vi "template-json-interface.vi"() -> ()   [LabVIEW 2024]
uses:
  template-state-machine-iwh/state-enum.ctl
  utils-sub-vi/csv-file-logging-util/filepath-selection.ctl
  utils-sub-vi/csv-file-logging-util/datalogging-options.ctl
  template-state-machine-iwh/serial-options.ctl
  template-state-machine-iwh/sensor-options.ctl
  <vilib>/Instr/_visa.llb/VISA Configure Serial Port (Instr).vi
  arduino-serial-ctrl.ctl
panel:
  out "Units":string
  out "Data":dbl
  out "Data Plot Chart":dbl(graph)
  out "Serial Port Open":bool
  out "Log File Open":bool
  in  "Tab Control":enum32{"Run", "Settings"}(tab)
  out "Logged CSV out":string
  out "Serial msg":string
  in  "Datalogging options":T1={"data-precision"=3, "Include Date"=FALSE, "Include Timestamp"=TRUE, "Include Milliseconds"=FALSE, "sample-rate (Hz)"=4.0, "Logging Active"=TRUE}
  in  "Log Filepath Selection":T2={"Log Filepath Source"=enum."Application Relative (Auto)", "Log File Path (Manual)"=path "C:/Users/dheard/Documents/0002-labview-projects/adam-4xxx/template/data", "Log File Folder Name"="data", "log file name"="log", "Include Date in Filename"=TRUE, "Include Time in Filename"=TRUE}
  in  "Serial Port Options":T3={"COM Port "="COM29", "baud rate (115200)"=115200, "Simulate Hardware"=FALSE} {"baud rate (115200)" max=115200 step=1200}
  in  "Sensor Options":T4={"Display Units"="PSI", "Zero Offset"=2.62, "Sensor Min"=0.0, "Sensor Max"=500.0, "Signal Min"=0.0, "Signal Max"=100.0, "Conversion Factor"=0.0}
  in  "save-settings":bool
  in  "load-settings":bool
  in  "Settings file":path=path "C:/Users/dheard/Documents/0002-labview-projects/labview-template-state-machine/settings/arduino-json-config.ini"
  out "Sample Rate (Hz)":dbl format="%-#3.3f"
  in  "Debug Mode":bool
  out "Loop Time (mS)":u32
  out "State:":T5
  out "error IO":errorcluster
  in  "stop":bool
  in  "start":bool
  in  "Exit":bool
  # "Arduino JSON Interface"
  # "Live Data"
  # "Conversion Factor to\nCalculate User Units from Sensor Units"
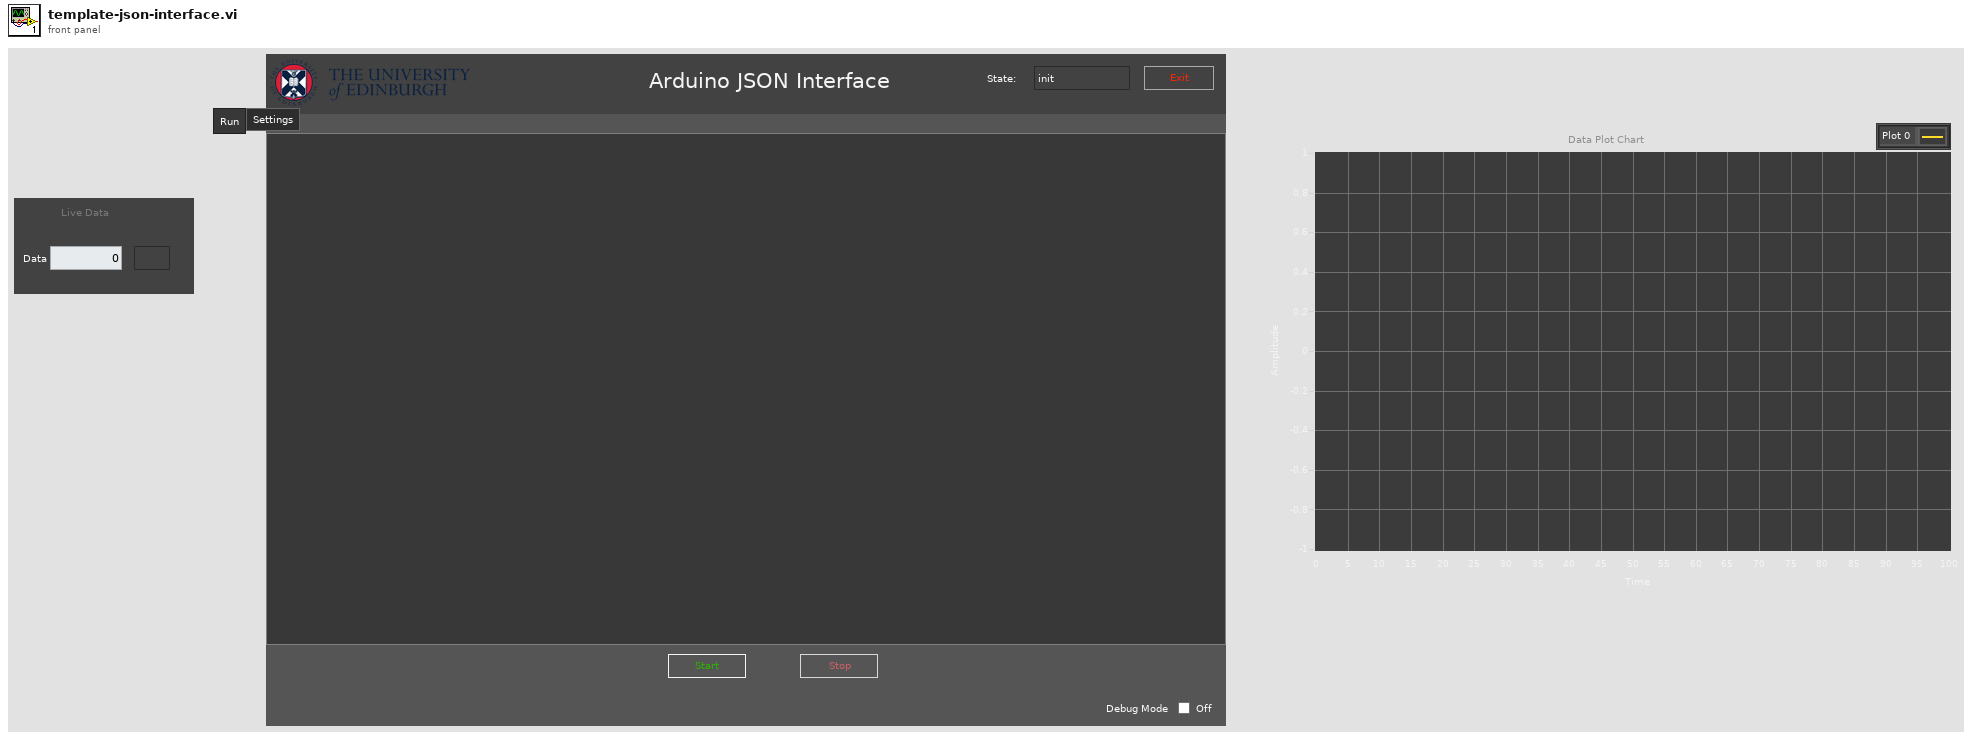
[diagram p1: front panel]
types:
  T1 = typedef "datalogging-options.ctl" = cluster{"data-precision":i32, "Include Date":bool, "Include Timestamp":bool, "Include Milliseconds":bool, "sample-rate (Hz)":dbl, "Logging Active":bool}
  T2 = typedef "filepath-selection.ctl" = cluster{"Log Filepath Source":enum16{"Application Relative (Auto)", "VI Relative (Auto)", "Complete Path (Manual)"}, "Log File Path (Manual)":path, "Log File Folder Name":string, "log file name":string, "Include Date in Filename":bool, "Include Time in Filename":bool}
  T3 = typedef "arduino-serial-ctrl.ctl" = cluster{"COM Port ":refnum<visa-resource-name>, "baud rate (115200)":u32, "Simulate Hardware":bool}
  T4 = typedef "sensor-options.ctl" = cluster{"Display Units":string, "Zero Offset":dbl, "Sensor Min":dbl, "Sensor Max":dbl, "Signal Min":dbl, "Signal Max":dbl, "Conversion Factor":dbl}
  T5 = typedef "state-enum.ctl" = enum16{"init", "recall-settings", "save-settings", "wait", "start", "pre-run", "run", "stop", "shutdown", "exit"}
  T6 = typedef "serial-options.ctl" = cluster{"COM Port (COM10)":refnum<visa-resource-name>, "baud rate (19200)":u32, "Simulate Hardware":bool}
  T7 = enum8{"Enabled", "Disabled", "Disabled and Grayed Out"}
  T8 = enum16{"open", "replace", "create", "open or create", "replace or create", "replace or create with confirmation"}
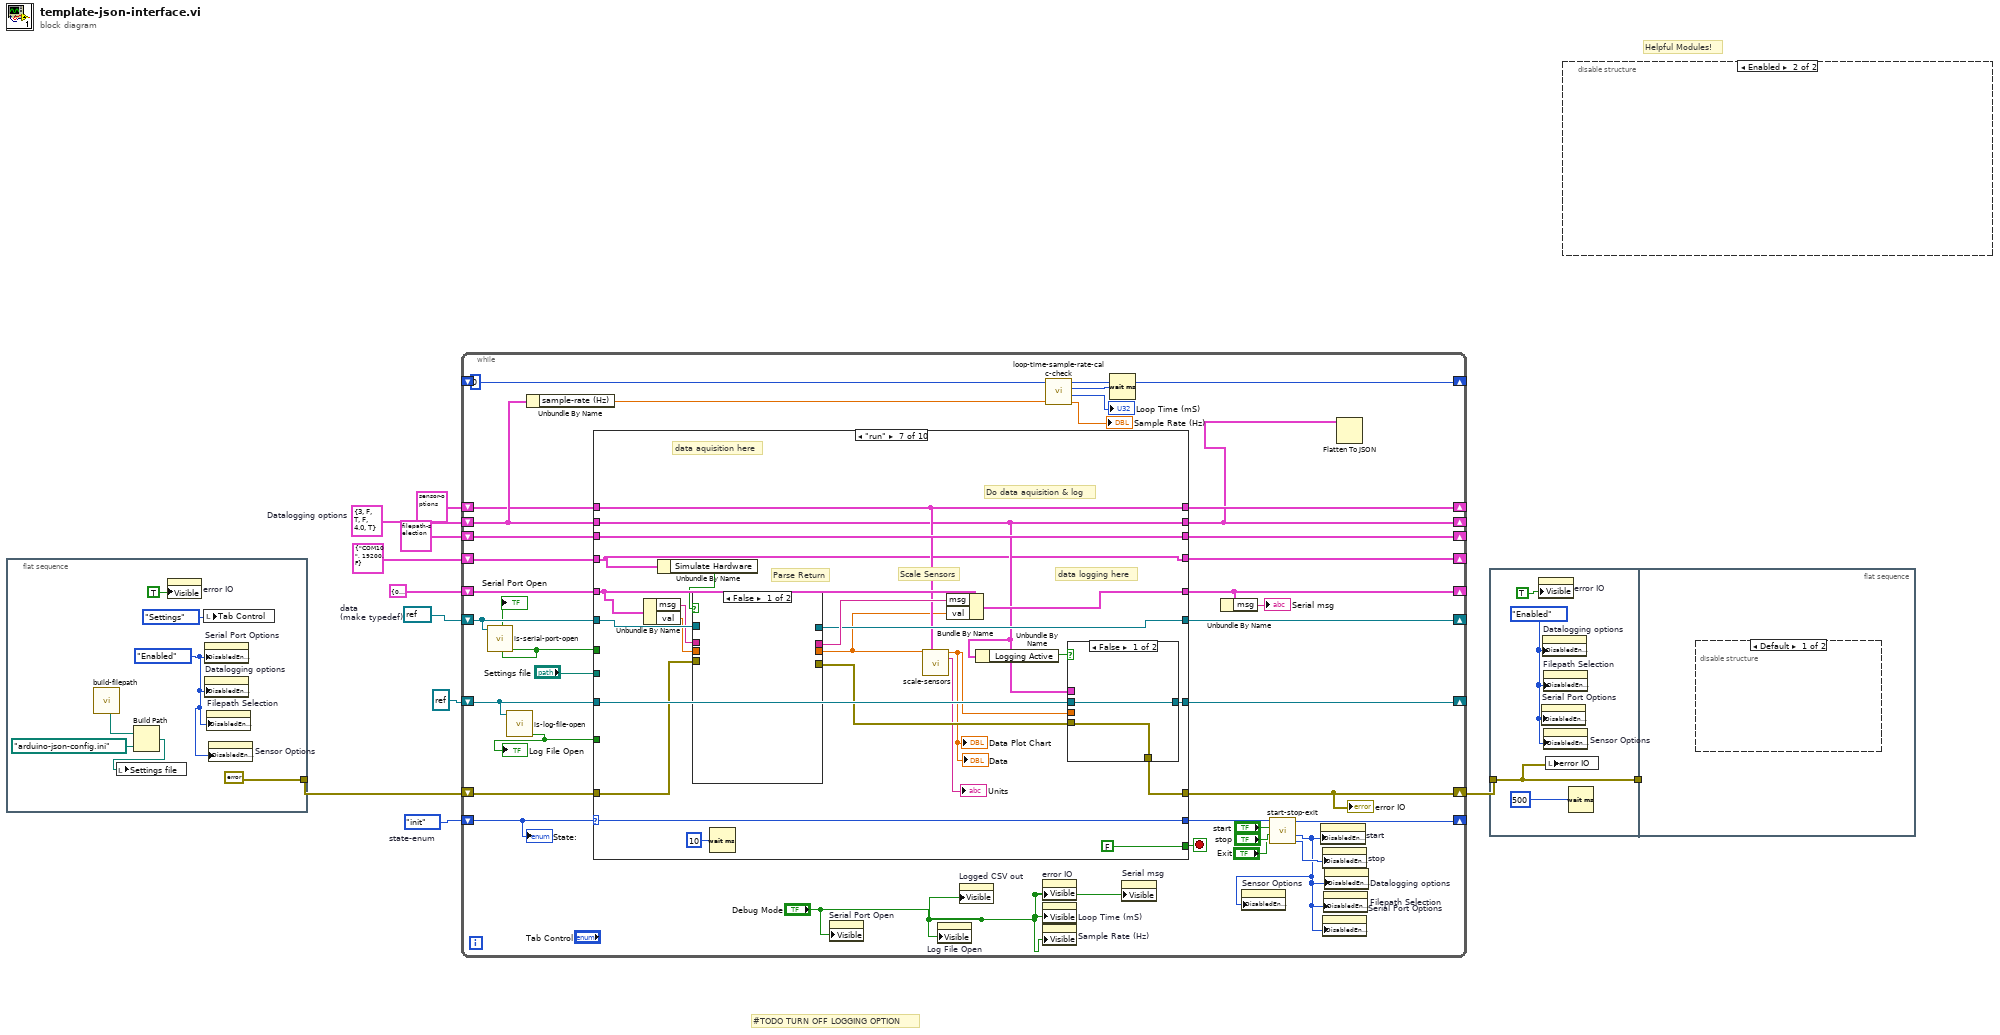
[diagram p0: block diagram]
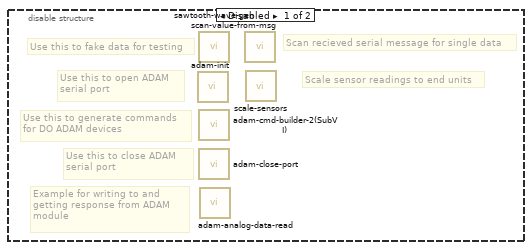
[diagram p2: hidden frame]
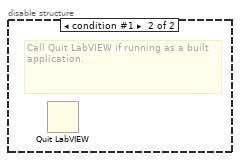
[diagram p3: hidden frame]
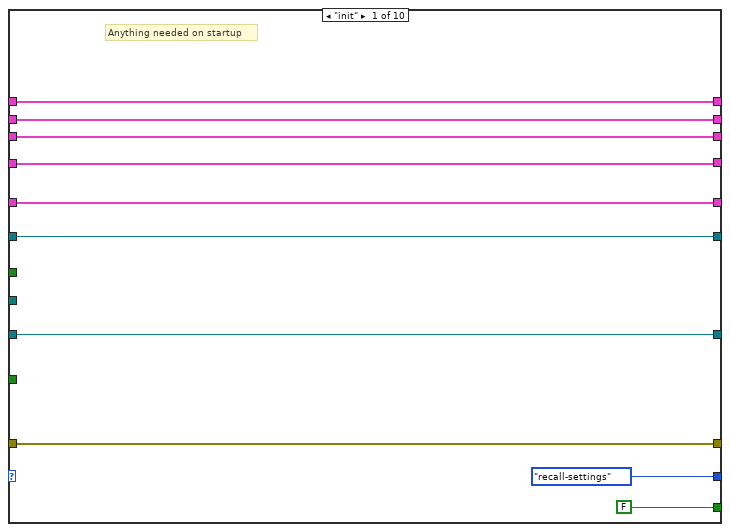
[diagram p4: hidden frame]
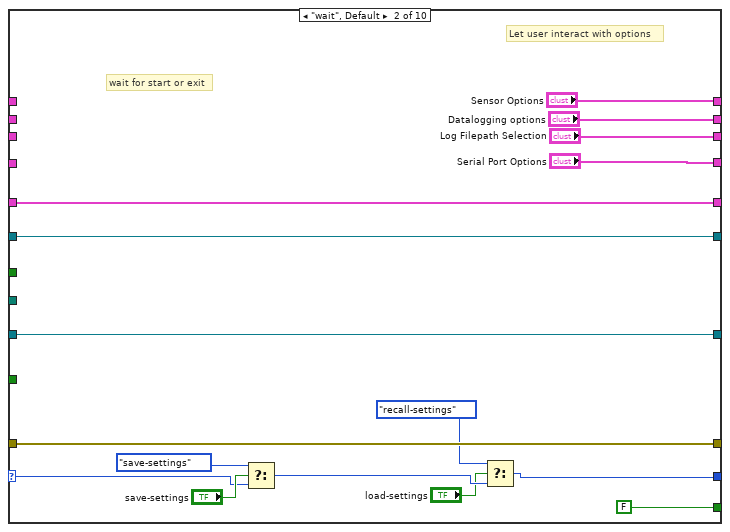
[diagram p5: hidden frame]
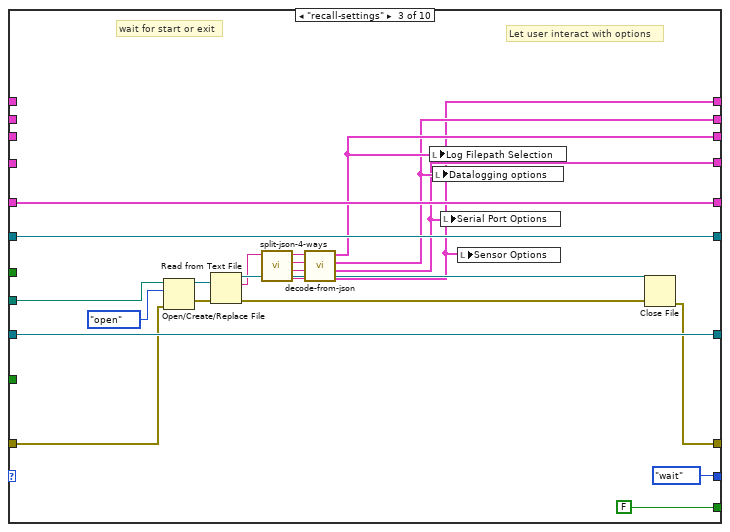
[diagram p6: hidden frame]
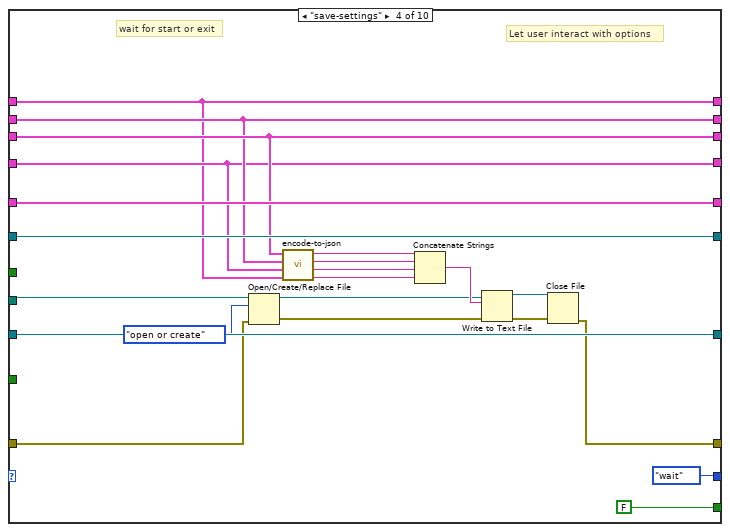
[diagram p7: hidden frame]
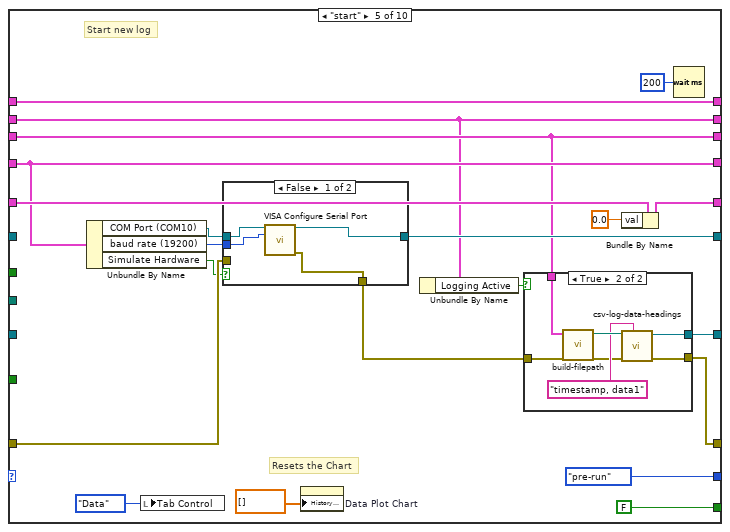
[diagram p8: hidden frame]
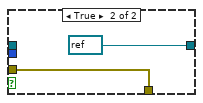
[diagram p9: hidden frame]
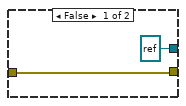
[diagram p10: hidden frame]
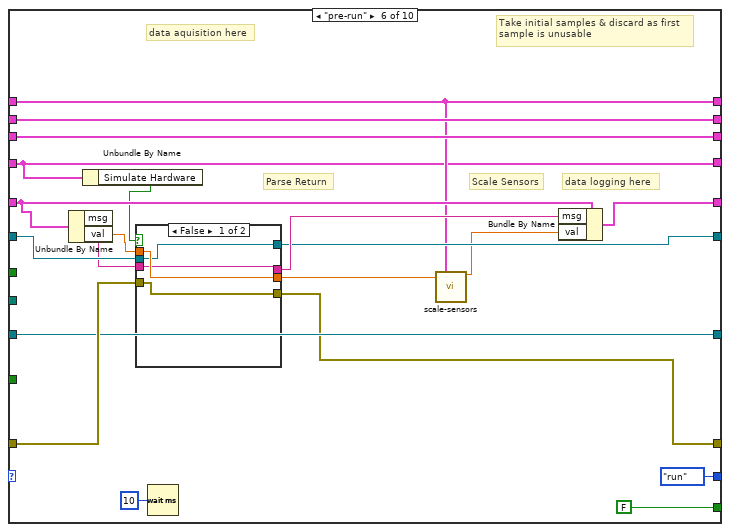
[diagram p11: hidden frame]
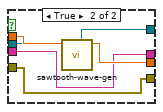
[diagram p12: hidden frame]
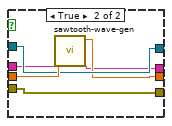
[diagram p13: hidden frame]
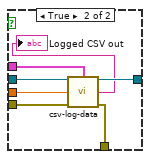
[diagram p14: hidden frame]
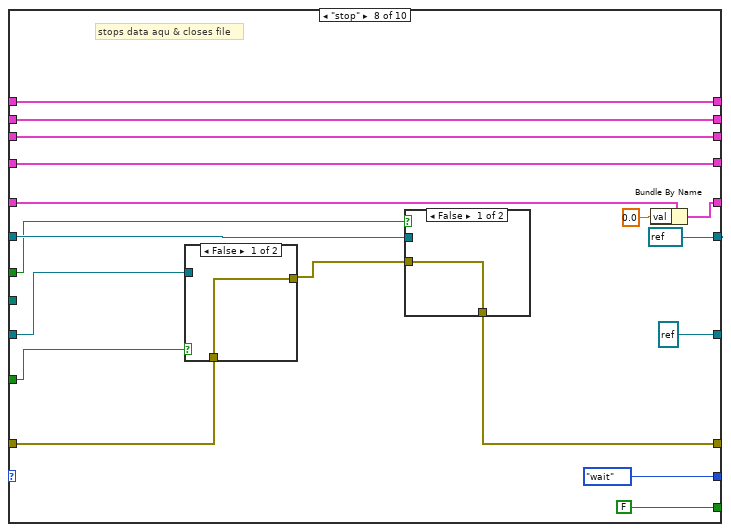
[diagram p15: hidden frame]
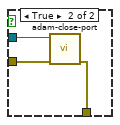
[diagram p16: hidden frame]
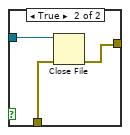
[diagram p17: hidden frame]
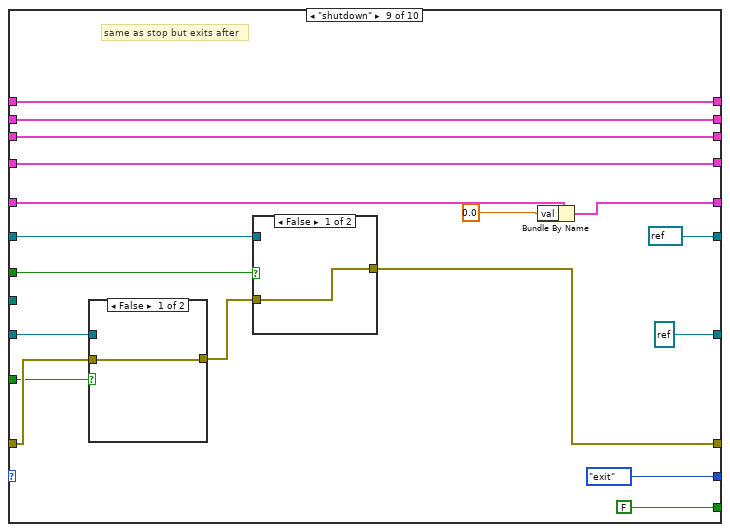
[diagram p18: hidden frame]
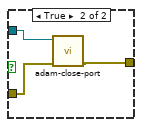
[diagram p19: hidden frame]
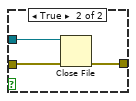
[diagram p20: hidden frame]
diagram:
  w4 = T1 {"data-precision"=3, "Include Date"=FALSE, "Include Timestamp"=TRUE, "Include Milliseconds"=FALSE, "sample-rate (Hz)"=4.0, "Logging Active"=TRUE}  # Datalogging options
  w9 = cluster{"val":dbl, "bool":bool, "msg":string} {"val"=0.0, "bool"=FALSE, "msg"=""}  # data (make typedef)
  w12 = state-enum."init"  # state-enum
  # "#TODO TURN OFF LOGGING OPTION"
  # "Helpful Modules!"
  n1 = flat-sequence {
    tunnel: [errorcluster {"status"=FALSE, "code"=0, "source"=""} ("error IO")] -> w8
    frame #0 {
      w16 = T7."Enabled" ("Disabled")
      n2 = call "build-filepath.vi"() -> ("Application Directory"=w15:path)  [unwired: 9 in, 2 out]
      n3 = Build Path(base path=w15, name or relative path=path "arduino-json-config.ini") -> (appended path=w13:path)
      n4 = local write "Settings file"(w13) -> ()
      n5 = property on="error IO" class="Clust (strict)"("Visible"=TRUE) -> ()  [unwired: 2 in, 2 out]
      n6 = local write "Tab Control"(enum32{"Data", "Settings"}."Settings" ("Tab Control")) -> ()
      n7 = property on="Serial Port Options" class="Clust (strict)"("DisabledEnum"=w16) -> ()  [unwired: 2 in, 2 out]
      n8 = property on="Datalogging options" class="Clust (strict)"("DisabledEnum"=w16) -> ()  [unwired: 2 in, 2 out]
      n9 = property on="Filepath Selection" class="Clust (strict)"("DisabledEnum"=w16) -> ()  [unwired: 2 in, 2 out]
      n10 = property on="Sensor Options" class="Clust (strict)"("DisabledEnum"=w16) -> ()  [unwired: 2 in, 2 out]
    }
  }
  n11 = while {
    shift-right: [w53] -> _
    shift-left: w12 -> [w55]
    shift-right: [w47] -> w10
    shift-left: w8 -> [w48]
    shift-right: [w28] -> _
    shift-left: w9 -> [w46]
    shift-right: [w43] -> _
    shift-left: u32 0 ("millisecond timer value") -> [w45]
    shift-right: [w39] -> _
    shift-left: T2 {"Log Filepath Source"=enum."Application Relative (Auto)", "Log File Path (Manual)"=path "C:/Users/dheard/Documents/0002-labview-projects/ammonia-absorbsion-rig/data", "Log File Folder Name"="data", "log file name"="log", "Include Date in Filename"=TRUE, "Include Time in Filename"=TRUE} ("Filepath Selection") -> [w38]
    shift-right: [w37] -> _
    shift-left: refnum<file> refnum ("Byte Stream File out") -> [w36]
    shift-right: [w21] -> _
    shift-left: w4 -> [w34]
    shift-right: [w31] -> _
    shift-left: T6 {"COM Port (COM10)"="COM10", "baud rate (19200)"=19200, "Simulate Hardware"=FALSE} ("Serial Port Options") -> [w32]
    shift-right: [w30] -> _
    shift-left: refnum<visa-resource-name> refnum ("VISA resource name out") -> [w29]
    shift-right: [w25] -> _
    shift-left: T4 {"Display Units"="units", "Zero Offset"=2.62, "Sensor Min"=0.0, "Sensor Max"=500.0, "Signal Min"=0.0, "Signal Max"=100.0, "Conversion Factor"=0.0} ("Sensor Options") -> [w23]
    stop <- w49 stop-if-true
    n12 = call "is-serial-port-open.vi"("VISA Refnum in"=w29) -> ("port-status"=w26:bool)  [unwired: 10 in]
    "Serial Port Open" <- w26
    n13 = call "is-log-file-open.vi"("Byte Stream File in"=w36) -> ("Log File Open"=w35:bool)  [unwired: 10 in]
    "Log File Open" <- w35
    n14 = Unbundle By Name(w34) -> ("sample-rate (Hz)"=w33:dbl)
    n15 = case shown="\"run\"" w55 {
      selector: w55 -> [_ w71 _ _ _ _ w212 _ _ _]
      tunnel: [state-enum."recall-settings" w66 state-enum."wait" state-enum."wait" state-enum."pre-run" state-enum."run" w212 state-enum."wait" state-enum."exit" state-enum."exit"] -> w54
      tunnel: [FALSE FALSE FALSE FALSE FALSE FALSE FALSE FALSE FALSE TRUE] -> w49
      tunnel: [w63 w80 w92 w104 w139 w166 w207 w231 w255 w287] -> w47
      tunnel: w48 -> [w63 w80 w96 w110 w133 w175 w205 w238 w264 w287]
      tunnel: [w62 w79 w102 w124 w143 w179 w211 w241 w267 w286] -> w28
      tunnel: w46 -> [w62 w79 w102 w124 w144 w173 w203 w243 w269 w286]
      tunnel: [w60 "Log Filepath Selection" w85 w117 w129 w178 w208 w237 w263 w284] -> w39
      tunnel: w38 -> [w60 _ _ w117 w129 w178 w208 w237 w263 w284]
      tunnel: [w61 w77 w101 w123 w140 w167 w209 refnum<file> refnum ("log file Byte Stream File out") refnum<file> refnum ("log file Byte Stream File out") w285] -> w37
      tunnel: w36 -> [w61 w77 w101 w123 _ w167 w210 w240 w266 w285]
      tunnel: [w59 "Datalogging options" w84 w116 w128 w177 w195 w236 w262 w283] -> w21
      tunnel: w34 -> [w59 _ _ w116 w128 w177 w195 w236 w262 w283]
      tunnel: w35 -> [_ _ _ _ _ _ _ w229 w261 _]
      tunnel: w32 -> [w58 _ _ w115 w137 w163 w193 w235 w260 w282]
      tunnel: [w58 "Serial Port Options" w83 w115 w137 w163 w193 w235 w260 w282] -> w31
      tunnel: [w57 w74 w100 w122 w134 w170 w199 refnum<visa-resource-name> refnum ("VISA resource name out") refnum<visa-resource-name> refnum ("VISA resource name out") w281] -> w30
      tunnel: w29 -> [w57 w74 w100 w122 _ w176 w206 w234 w258 w281]
      tunnel: w26 -> [_ _ _ _ _ _ _ w228 w259 _]
      tunnel: [w56 "Sensor Options" w82 w114 w131 w169 w198 w230 w254 w280] -> w25
      tunnel: w23 -> [w56 _ _ w114 w131 w169 w198 w230 w254 w280]
      tunnel: "Settings file" -> [_ _ w98 w105 _ _ _ _ _ _]
      frame "init" {
        # "Anything needed on startup"
      }
      frame "wait", Default {
        # "Let user interact with options"
        # "wait for start or exit"
        n16 = Select(t=state-enum."save-settings", s="save-settings", f=w71) -> (s? t:f=w69:T5)
        n17 = Select(t=state-enum."recall-settings", s="load-settings", f=w69) -> (s? t:f=w66:T5)
      }
      frame "recall-settings" {
        # "Let user interact with options"
        # "wait for start or exit"
        n18 = Open/Create/Replace File(file path (use dialog)=w98, error in=w96, operation (0:open)=T8."open") -> (refnum out=w95:refnum<file>, error out=w94:errorcluster)  [unwired: 3 in, 1 out]
        n19 = Read from Text File(file (use dialog)=w95, error in=w94) -> (refnum out=w91:refnum<file>, text=w90:string, error out=w93:errorcluster)  [unwired: 2 in, 1 out]
        n20 = call "split-json-4-ways.vi"("json-string-in"=w90) -> ("sensor-json"=w86:string, "serial-json"=w87:string, "datalogging-json"=w88:string, "filepath-json"=w89:string)  [unwired: 7 in]
        n21 = call "decode-from-json.vi"("sensor-options-json"=w86, "serial-port-json"=w87, "data-logging-json"=w88, "filepath-json"=w89) -> ("Sensor Option Recall"=w82:T4, "Serial Port Recall"=w83:T6, "Datalogging Recall"=w84:T1, "Filepath Recall"=w85:T2)  [unwired: 4 in]
        n22 = local write "Log Filepath Selection"(w85) -> ()
        n23 = local write "Datalogging options"(w84) -> ()
        n24 = local write "Serial Port Options"(w83) -> ()
        n25 = local write "Sensor Options"(w82) -> ()
        n26 = Close File(refnum=w91, error in=w93) -> (error out=w92:errorcluster)  [unwired: 1 out]
      }
      frame "save-settings" {
        # "Let user interact with options"
        # "wait for start or exit"
        n27 = Open/Create/Replace File(file path (use dialog)=w105, error in=w110, operation (0:open)=T8."open or create") -> (refnum out=w109:refnum<file>, error out=w108:errorcluster)  [unwired: 3 in, 1 out]
        n28 = call "encode-to-json.vi"("Sensor Options"=w114, "Serial Port Options"=w115, "Datalogging options"=w116, "Filepath Selection"=w117) -> ("sensor-options-json"=w113:string, "serial-port-json"=w118:string, "data-logging-json"=w119:string, "filepath-json"=w120:string)  [unwired: 4 in]
        n29 = Concatenate Strings(w120, w119, w118, w113) -> (w112:string)
        n30 = Write to Text File(file (use dialog)=w109, text=w112, error in=w108) -> (refnum out=w107:refnum<file>, error out=w106:errorcluster)  [unwired: 1 in, 1 out]
        n31 = Close File(refnum=w107, error in=w106) -> (error out=w104:errorcluster)  [unwired: 1 out]
      }
      frame "start" {
        # "Start new log"
        # "Resets the Chart"
        n32 = Unbundle By Name(w137) -> ("COM Port (COM10)"=w136:refnum<visa-resource-name>, "baud rate (19200)"=w135:u32, "Simulate Hardware"=w126:bool)
        n33 = local write "Tab Control"(enum32{"Data", "Settings"}."Data" ("Tab Control")) -> ()
        n34 = case shown="False" w126 {
          tunnel: w136 -> [w150 _]
          tunnel: w135 -> [w149 _]
          tunnel: [w148 refnum<visa-resource-name> refnum ("VISA resource name out")] -> w134
          tunnel: w133 -> [_ w151]
          tunnel: [w147 w151] -> w132
          frame False {
            n35 = call-poly "VISA Configure Serial Port"("VISA resource name"=w150, "baud rate (9600)"=w149) -> ("VISA resource name out"=w148:refnum<visa-resource-name>, "error out"=w147:errorcluster)  [unwired: 12 in]
          }
          frame True {
          }
        }
        n36 = property on="Data Plot Chart" class="WFChart (strict)"("History Data"=dbl[] []) -> ()  [unwired: 2 in, 2 out]
        n37 = Unbundle By Name(w128) -> ("Logging Active"=w127:bool)
        n38 = case shown="True" w127 {
          tunnel: [refnum<file> refnum ("Byte Stream File out") w158] -> w140
          tunnel: [w153 w157] -> w139
          tunnel: w132 -> [w153 w156]
          tunnel: w129 -> [_ w155]
          frame False {
          }
          frame True {
            n39 = call "build-filepath.vi"("Filepath Selection"=w155) -> ("appended path for log file"=w160:path)  [unwired: 8 in, 2 out]
            n40 = call "csv-log-data-headings.vi"("CSV Data Headings"="timestamp, data1", "error in (no error)"=w156, "Log File Path"=w160) -> ("error out"=w157:errorcluster, "Byte Stream File out"=w158:refnum<file>)  [unwired: 6 in, 1 out]
          }
        }
        n41 = Bundle By Name(cluster=w144, "val"=0.0 ("output")) -> (w143:cluster{"val":dbl, "bool":bool, "msg":string})
        n42 = Wait (ms)(milliseconds to wait=u32 200) -> ()  [unwired: 1 out]
      }
      frame "pre-run" {
        # "Take initial samples & discard as first\nsample is unusable"
        # "Scale Sensors"
        # "Parse Return"
        # "data logging here"
        # "data aquisition here"
        n43 = Unbundle By Name(w173) -> ("msg"=w172:string, "val"=w161:dbl)
        n44 = Unbundle By Name(w163) -> ("Simulate Hardware"=w162:bool)
        n45 = case shown="False" w162 {
          tunnel: w176 -> [w181 w185]
          tunnel: w175 -> [w184 w186]
          tunnel: w172 -> [w182 w187]
          tunnel: [w182 w187] -> w171
          tunnel: [w181 w185] -> w170
          tunnel: [w183 w188] -> w168
          tunnel: [w184 w186] -> w166
          tunnel: w161 -> [w183 w189]
          frame False {
          }
          frame True {
            n46 = call "sawtooth-wave-gen.vi"("current-val"=w189) -> ("output"=w188:dbl)  [unwired: 10 in]
          }
        }
        n47 = Wait (ms)(milliseconds to wait=u32 10) -> ()  [unwired: 1 out]
        n48 = call "scale-sensors.vi"("Measured Value (mV)"=w168, "Sensor Options"=w169) -> ("Calculated Value (User Specified Unit)"=w164:dbl)  [unwired: 8 in, 5 out]
        n49 = Bundle By Name(cluster=w173, "msg"=w171, "val"=w164) -> (w179:cluster{"val":dbl, "bool":bool, "msg":string})
      }
      frame "run" {
        # "Scale Sensors"
        # "Parse Return"
        # "data logging here"
        # "data aquisition here"
        # "Do data aquisition & log"
        n50 = Unbundle By Name(w203) -> ("msg"=w202:string, "val"=w191:dbl)
        n51 = Unbundle By Name(w193) -> ("Simulate Hardware"=w192:bool)
        n52 = case shown="False" w192 {
          tunnel: w206 -> [_ w216]
          tunnel: w205 -> [_ w218]
          tunnel: w202 -> [_ w214]
          tunnel: [_ w218] -> w201
          tunnel: [_ w214] -> w200
          tunnel: [_ w216] -> w199
          tunnel: [_ w215] -> w190
          tunnel: w191 -> [_ w217]
          frame False {
          }
          frame True {
            n53 = call "sawtooth-wave-gen.vi"("current-val"=w217) -> ("output"=w215:dbl)  [unwired: 10 in]
          }
        }
        n54 = Wait (ms)(milliseconds to wait=u32 10) -> ()  [unwired: 1 out]
        n55 = call "scale-sensors.vi"("Measured Value (mV)"=w190, "Sensor Options"=w198) -> ("Calculated Value (User Specified Unit)"=w197:dbl, "Display Units"=→"Units":string)  [unwired: 8 in, 4 out]
        "Data" <- w197
        "Data Plot Chart" <- w197
        n56 = Bundle By Name(cluster=w203, "msg"=w200, "val"=w190) -> (w211:cluster{"val":dbl, "bool":bool, "msg":string})
        n57 = Unbundle By Name(w195) -> ("Logging Active"=w194:bool)
        n58 = case shown="False" w194 {
          tunnel: w210 -> [w220 w227]
          tunnel: [w220 w226] -> w209
          tunnel: [w219 w224] -> w207
          tunnel: w195 -> [_ w223]
          tunnel: w201 -> [w219 w222]
          tunnel: w197 -> [_ w221]
          frame False {
          }
          frame True {
            n59 = call "csv-log-data.vi"("log file Byte Stream File in"=w227, "Datalogging options"=w223, "Data Point In"=w221, "error in (no error)"=w222) -> ("log file Byte Stream File out"=w226:refnum<file>, "Logged CSV out"=→"Logged CSV out":string, "error out"=w224:errorcluster)  [unwired: 7 in, 2 out]
          }
        }
      }
      frame "stop" {
        # "stops data aqu & closes file"
        n60 = case shown="False" w229 {
          tunnel: w240 -> [_ w253]
          tunnel: w238 -> [w250 w252]
          tunnel: [w250 w251] -> w232
          frame False {
          }
          frame True {
            n61 = Close File(refnum=w253, error in=w252) -> (error out=w251:errorcluster)  [unwired: 1 out]
          }
        }
        n62 = case shown="False" w228 {
          tunnel: w234 -> [_ w249]
          tunnel: w232 -> [w246 w248]
          tunnel: [w246 w247] -> w231
          frame False {
          }
          frame True {
            n63 = call "adam-close-port.vi"("error in (no error)"=w248, "VISA Refnum in"=w249) -> ("error out"=w247:errorcluster)  [unwired: 9 in]
          }
        }
        n64 = Bundle By Name(cluster=w243, "val"=0.0 ("output")) -> (w241:cluster{"val":dbl, "bool":bool, "msg":string})
      }
      frame "shutdown" {
        # "same as stop but exits after"
        n65 = case shown="False" w261 {
          tunnel: w266 -> [_ w279]
          tunnel: w264 -> [w276 w278]
          tunnel: [w276 w277] -> w256
          frame False {
          }
          frame True {
            n66 = Close File(refnum=w279, error in=w278) -> (error out=w277:errorcluster)  [unwired: 1 out]
          }
        }
        n67 = case shown="False" w259 {
          tunnel: w258 -> [_ w275]
          tunnel: w256 -> [w272 w274]
          tunnel: [w272 w273] -> w255
          frame False {
          }
          frame True {
            n68 = call "adam-close-port.vi"("error in (no error)"=w274, "VISA Refnum in"=w275) -> ("error out"=w273:errorcluster)  [unwired: 9 in]
          }
        }
        n69 = Bundle By Name(cluster=w269, "val"=0.0 ("output")) -> (w267:cluster{"val":dbl, "bool":bool, "msg":string})
      }
      frame "exit" {
        # "Exit safely"
      }
    }
    "error IO" <- w47
    n70 = property on="Serial Port Open" class="Bool (strict)"("Visible"="Debug Mode") -> ()  [unwired: 2 in, 2 out]
    n71 = property on="Log File Open" class="Bool (strict)"("Visible"="Debug Mode") -> ()  [unwired: 2 in, 2 out]
    n72 = property on="Logged CSV out" class="Str"("Visible"="Debug Mode") -> ()  [unwired: 2 in, 2 out]
    n73 = property on="error IO" class="Clust (strict)"("Visible"="Debug Mode") -> ()  [unwired: 2 in, 2 out]
    n74 = property on="Loop Time (mS)" class="DigNum (strict)"("Visible"="Debug Mode") -> ()  [unwired: 2 in, 2 out]
    n75 = property on="Sample Rate (Hz)" class="DigNum (strict)"("Visible"="Debug Mode") -> ()  [unwired: 2 in, 2 out]
    n76 = call "loop-time-sample-rate-calc-check.vi"("sample-rate-Hz"=w33, "millisecond timer value in"=w45) -> ("Loop Hz"=→"Sample Rate (Hz)":dbl, "Loop Time (mS)"=→"Loop Time (mS)":u32, "sample-rate-delay-mS"=w40:u32, "millisecond timer value out"=w43:u32)  [unwired: 6 in]
    n77 = Wait (ms)(milliseconds to wait=w40) -> ()  [unwired: 1 out]
    n78 = property on="Serial msg" class="Str"("Visible"="Debug Mode") -> ()  [unwired: 2 in, 2 out]
    n79 = Unbundle By Name(w28) -> ("msg"=→"Serial msg":string)
    n80 = call "start-stop-exit.vi"("Exit"="Exit", "stop"="stop", "start"="start", "current-state"=w54) -> ("stop-enable"=w44:T7, "start-enable"=w24:T7, "new-state"=w53:T5)  [unwired: 5 in]
    n81 = property on="Sensor Options" class="Clust (strict)"("DisabledEnum"=w24) -> ()  [unwired: 2 in, 2 out]
    n82 = property on="start" class="Bool"("DisabledEnum"=w24) -> ()  [unwired: 2 in, 2 out]
    n83 = property on="stop" class="Bool"("DisabledEnum"=w44) -> ()  [unwired: 2 in, 2 out]
    n84 = property on="Serial Port Options" class="Clust (strict)"("DisabledEnum"=w24) -> ()  [unwired: 2 in, 2 out]
    n85 = property on="Filepath Selection" class="Clust (strict)"("DisabledEnum"=w24) -> ()  [unwired: 2 in, 2 out]
    n86 = property on="Datalogging options" class="Clust (strict)"("DisabledEnum"=w24) -> ()  [unwired: 2 in, 2 out]
    n87 = Flatten To JSON(anything=w21) -> ()  [unwired: 2 in, 2 out]
    "State:" <- w55
  }
  n88 = flat-sequence {
    tunnel: [w291] -> w11
    tunnel: w10 -> [w291]
    tunnel: w11 -> [_]
    frame #0 {
      w290 = T7."Enabled" ("Disabled")
      n89 = property on="error IO" class="Clust (strict)"("Visible"=TRUE) -> ()  [unwired: 2 in, 2 out]
      n90 = property on="Serial Port Options" class="Clust (strict)"("DisabledEnum"=w290) -> ()  [unwired: 2 in, 2 out]
      n91 = property on="Datalogging options" class="Clust (strict)"("DisabledEnum"=w290) -> ()  [unwired: 2 in, 2 out]
      n92 = property on="Filepath Selection" class="Clust (strict)"("DisabledEnum"=w290) -> ()  [unwired: 2 in, 2 out]
      n93 = property on="Sensor Options" class="Clust (strict)"("DisabledEnum"=w290) -> ()  [unwired: 2 in, 2 out]
      n94 = local write "error IO"(w291) -> ()
      n95 = Wait (ms)(milliseconds to wait=u32 500) -> ()  [unwired: 1 out]
    }
    frame #1 {
      n96 = disable-structure "Conditional Disable Structure" shown="Default" {
        frame condition #0 (active) {
        }
        frame condition #1 {
          # "Call Quit LabVIEW if running as a built application."
          n97 = Quit LabVIEW() -> ()  [unwired: 1 in]
        }
      }
    }
  }
  n98 = disable-structure shown="Enabled" {
    frame Disabled {
      # "Scale sensor readings to end units"
      # "Scan recieved serial message for single data"
      # "Example for writing to and\ngetting response from ADAM\nmodule"
      # "Use this to open ADAM\nserial port"
      # "Use this to close ADAM \nserial port"
      # "Use this to generate commands\nfor DO ADAM devices"
      # "Use this to fake data for testing"
      n99 = call "adam-init.vi"() -> ()  [unwired: 10 in, 2 out]
      n100 = call "sawtooth-wave-gen.vi"() -> ()  [unwired: 11 in, 1 out]
      n101 = call "adam-cmd-builder-2(SubVI).vi"() -> ()  [unwired: 6 in, 6 out]
      n102 = call "adam-close-port.vi"() -> ()  [unwired: 11 in, 1 out]
      n103 = call "adam-analog-data-read.vi"() -> ()  [unwired: 7 in, 5 out]
      n104 = call "scan-value-from-msg.vi"() -> ()  [unwired: 9 in, 3 out]
      n105 = call "scale-sensors.vi"() -> ()  [unwired: 10 in, 6 out]
    }
    frame Enabled {
    }
  }
